vi "Parse Info Section.vi"(8 "error in":errorcluster, 11 "reference in":refnum<class "Electronic Datasheet.lvclass">) -> (0 "error out":errorcluster, 3 "reference out":refnum<class "Electronic Datasheet.lvclass">)   [LabVIEW 2020, in "Electronic Datasheet.lvlib" / "Electronic Datasheet.lvclass"]
uses:
  Electronic Datasheet.lvclass
  Core/Device Info/Device Info.lvclass
  Core/File Info/File Info.lvclass
  Core/Info Section/Info Section.lvclass
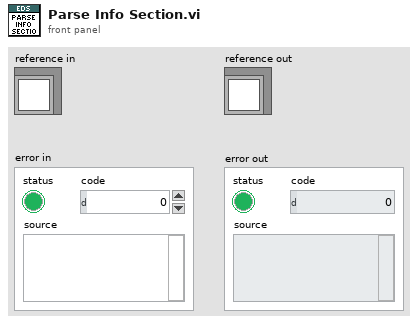
[diagram p1: front panel]
types:
  T1 = typedef "Electronic Datasheet.lvlib/Electronic Datasheet.lvclass/ObjectAttributes.ctl" = cluster{"EDS File Path":path, "Object Dict":refnum<class "Dictionary.lvclass">, "Sorted Object Dict":refnum<class "Sorted Object Dictionary.lvclass">, "Device Info":refnum<class "Device Info.lvclass">, "File Info":refnum<class "File Info.lvclass">}
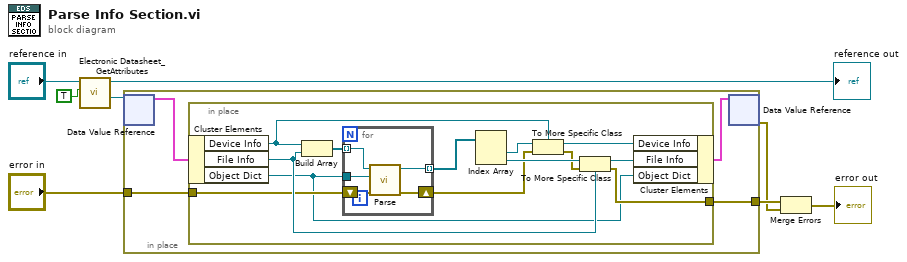
[diagram p0: block diagram]
diagram:
  n1 = call "Electronic Datasheet_GetAttributes.vi"("OnlyGetDvrReference(False)"=TRUE, "reference in"="reference in") -> ("DataRef"=w3:refnum<data-value>, "reference out"=→"reference out":refnum<class "Electronic Datasheet.lvclass">)  [unwired: 6 in, 2 out]
  n2 = in-place {
    in-place-border: [w10] -> w8
    in-place-border: "error in" -> [w11]
    n3 = in-place-dvr #1(w3) -> (w12:T1)  [unwired: 1 out]
    n4 = in-place {
      in-place-border: [w25] -> w10
      in-place-border: w11 -> [w16]
      n5 = in-place-cluster #2(w12) -> ("Device Info"=w18:refnum<class "Device Info.lvclass">, "File Info"=w17:refnum<class "File Info.lvclass">, "Object Dict"=w13:refnum<class "Dictionary.lvclass">)
      n6 = Build Array(w18, w17) -> (w23:refnum<class "Info Section.lvclass">[])
      n7 = for {
        tunnel: [w29] -> w24 mode=indexing
        tunnel: w13 -> [w28]
        shift-right: [w30] -> w20
        shift-left: w16 -> [w27]
        tunnel: w23 -> [w26] mode=indexing
        n8 = call-dynamic "Parse.vi"("error in"=w27, "Object Dictionary"=w28, "Info Section in"=w26) -> ("error out"=w30:errorcluster, "Info Section out"=w29:refnum<class "Info Section.lvclass">)  [unwired: 7 in]
      }
      n9 = Index Array(array=w24) -> (element #1=w21:refnum<class "Info Section.lvclass">, element #2=w22:refnum<class "Info Section.lvclass">)  [unwired: 2 in]
      n10 = To More Specific Class(target class=w18, reference=w21, error in=w20) -> (specific class reference=w15:refnum<class "Device Info.lvclass">, error out=w19:errorcluster)
      n11 = To More Specific Class(target class=w17, reference=w22, error in=w19) -> (specific class reference=w14:refnum<class "File Info.lvclass">, error out=w25:errorcluster)
      n12 = in-place-cluster #2("Device Info"=w15, "File Info"=w14, "Object Dict"=w13) -> (w9:T1)
    }
    n13 = in-place-dvr #1(w9) -> (w1:errorcluster)  [unwired: 1 out]
  }
  n14 = Merge Errors(w8, w1) -> (→"error out":errorcluster)
